vi "Create Path Object.vi"(10 "Error In":errorcluster, 11 "Path Data Cluster":T1) -> (2 "Error Out":errorcluster, 3 "Path .NET Ref":refnum<k24>)   [LabVIEW 2015, in "VeriStand XML Parser.lvlib"]
doc: "Creates a Path .NET Object based off the path data cluster provided"
uses:
  VeriStand XML Parser.lvlib
  NationalInstruments.VeriStand.XMLReader
  XML Controls/Path Cluster.ctl
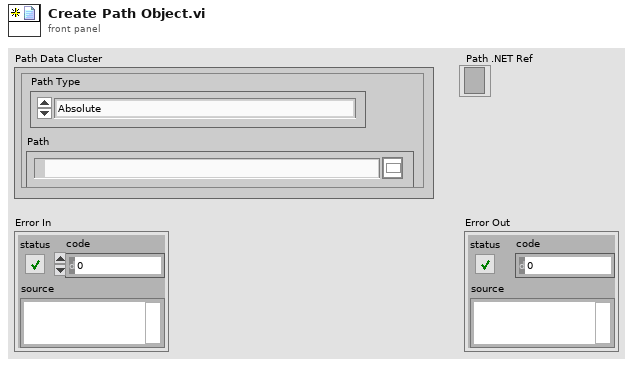
[diagram p1: front panel]
types:
  T1 = typedef "VeriStand XML Parser.lvlib/Path Cluster.ctl" = cluster{"Path":path, "Path Type":enum16{"Absolute", "To Base", "To Common Doc Dir", "To Application Data Dir"}}
  T2 = enum16{"Absolute", "To Base", "To Common Doc Dir", "To Application Data Dir"}
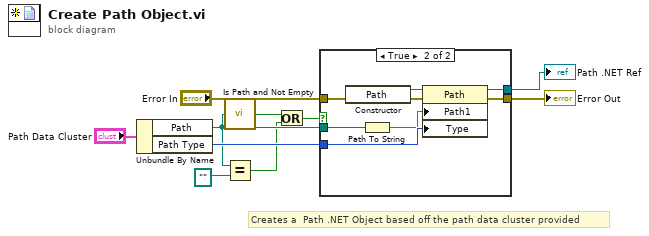
[diagram p0: block diagram]
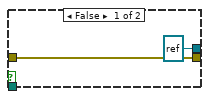
[diagram p2: hidden frame]
diagram:
  # "Creates a  Path .NET Object based off the path data cluster provided"
  n1 = Unbundle By Name("Path Data Cluster") -> ("Path"=w4:path, "Path Type"=w7:T2)
  n2 = call <vilib>:"Is Path and Not Empty.vi"("path"=w4) -> ("Is Path and Not Empty?"=w3:bool)  [unwired: 4 in]
  n3 = Equal?(x=w4, y=path "" ("path")) -> (x = y?=w2:bool)
  n4 = Or(x=w3, y=w2) -> (x .or. y?=w1:bool)
  n5 = case shown="True" w1 {
    tunnel: "Error In" -> [w12 w20]
    tunnel: [refnum<k24> refnum ("new reference") w19] -> w9
    tunnel: [w12 w18] -> w8
    tunnel: w7 -> [_ w17]
    tunnel: w4 -> [_ w16]
    frame False {
    }
    frame True {
      n6 = constructor class="Path"(error in=w20) -> (reference out=w14:refnum<k24>, error out=w13:errorcluster)  [unwired: 2 in, 1 out]
      n7 = Path To String(path=w16) -> (string=w15:string)
      n8 = property class="Path"(reference=w14, error in=w13, "Path1"=w15, "Type"=w17) -> (reference out=w19:refnum<k24>, error out=w18:errorcluster)
    }
  }
  "Path .NET Ref" <- w9
  "Error Out" <- w8
